vi "计算局面所有可能的走法（黑）.vi"(1 "输入的棋盘":T2) -> (0 "可能移动":T1(array[cluster]))   [LabVIEW 2017]
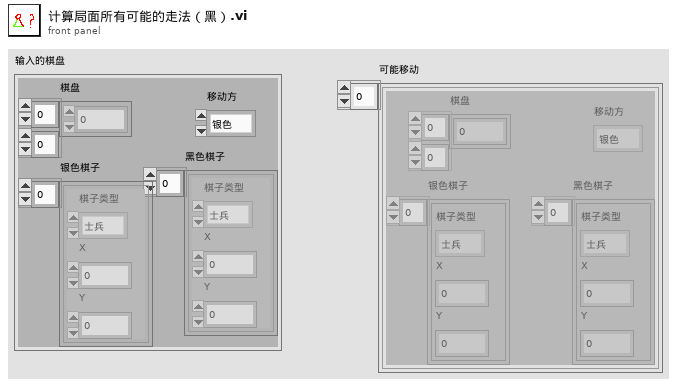
[diagram p1: front panel]
types:
  T1 = cluster{"棋盘":u16[][], "银色棋子":cluster{"棋子类型":enum16{"士兵", "骑士", "主教", "战车", "皇后", "国王", "空"}, "X":u8, "Y":u8}[], "黑色棋子":cluster{"棋子类型":enum16{"士兵", "骑士", "主教", "战车", "皇后", "国王", "空"}, "X":u8, "Y":u8}[], "移动方":enum16{"银色", "黑色"}}[]
  T2 = cluster{"棋盘":u16[][], "银色棋子":cluster{"棋子类型":enum16{"士兵", "骑士", "主教", "战车", "皇后", "国王", "空"}, "X":u8, "Y":u8}[], "黑色棋子":cluster{"棋子类型":enum16{"士兵", "骑士", "主教", "战车", "皇后", "国王", "空"}, "X":u8, "Y":u8}[], "移动方":enum16{"银色", "黑色"}}
  T3 = cluster{"棋子类型":enum16{"士兵", "骑士", "主教", "战车", "皇后", "国王", "空"}, "X":u8, "Y":u8}[]
  T4 = cluster{"棋子类型":enum16{"士兵", "骑士", "主教", "战车", "皇后", "国王", "空"}, "X":u8, "Y":u8}
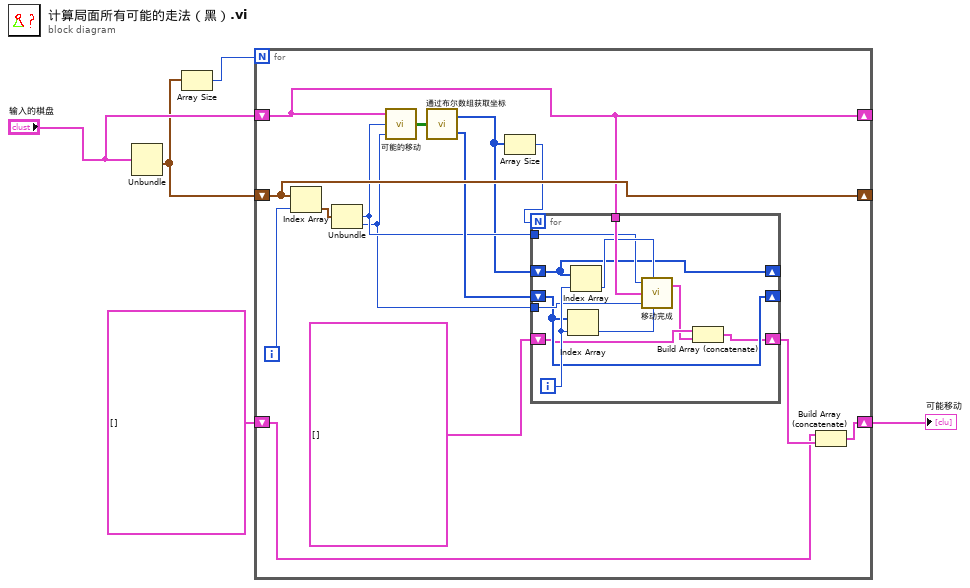
[diagram p0: block diagram]
diagram:
  n1 = Unbundle("输入的棋盘") -> ("黑色棋子"=w3:T3)  [unwired: 3 out]
  n2 = Array Size(array=w3) -> (size(s)=w4:i32)
  n3 = for {
    N: w4 -> [_]
    shift-right: [w14] -> _
    shift-left: "输入的棋盘" -> [w14]
    shift-right: [w17] -> _
    shift-left: w3 -> [w17]
    shift-right: [w8] -> w1
    shift-left: T1 [] -> [w9]
    i -> [w19]
    n4 = Index Array(array=w17, index=w19) -> (element=w18:T4)
    n5 = Unbundle(w18) -> ("X"=w13:u8, "Y"=w12:u8)  [unwired: 1 out]
    n6 = call "可能的移动.vi"("Y"=w12, "X"=w13, "游戏"=w14) -> ("输出数组"=w16:bool[][])
    n7 = call "通过布尔数组获取坐标.vi"("数组"=w16) -> ("X"=w7:i32[], "Y"=w15:i32[])
    n8 = Array Size(array=w7) -> (size(s)=w6:i32)
    n9 = for {
      N: w6 -> [_]
      shift-right: [w24] -> _
      shift-left: w7 -> [w24]
      shift-right: [w23] -> _
      shift-left: w15 -> [w23]
      tunnel: w14 -> [w30]
      tunnel: w13 -> [w26]
      tunnel: w12 -> [w25]
      shift-right: [w20] -> w10
      shift-left: T1 [] -> [w22]
      i -> [w29]
      n10 = Index Array(array=w23, index=w29) -> (element=w27:i32)
      n11 = Index Array(array=w24, index=w29) -> (element=w28:i32)
      n12 = call "移动完成.vi"("原始X"=w26, "移动后的X"=w28, "输入的棋盘"=w30, "原始Y"=w25, "移动后的Y"=w27) -> ("输出的棋盘"=w21:T2)  [unwired: 1 out]
      n13 = Build Array (concatenate)(w22, w21) -> (w20:T1)
    }
    n14 = Build Array (concatenate)(w9, w10) -> (w8:T1)
  }
  "可能移动" <- w1
